vi "Example_Cursor.vi"() -> ()   [LabVIEW 2020, in "LcPictureBox.lvclass"]
uses:
  LcPictureBox.lvclass
  System.Windows.Forms
  SmoothingMode.ctl
  Pen.ctl
  CursorType.ctl
  ce328d88-1fef-4cb5-b4df-921596365a82.vi
  2765cc97-931e-4dce-9eb0-820734866045.vi
panel:
  in  "PictureBox 1":refnum<k24>(container)
  out "error out":errorcluster
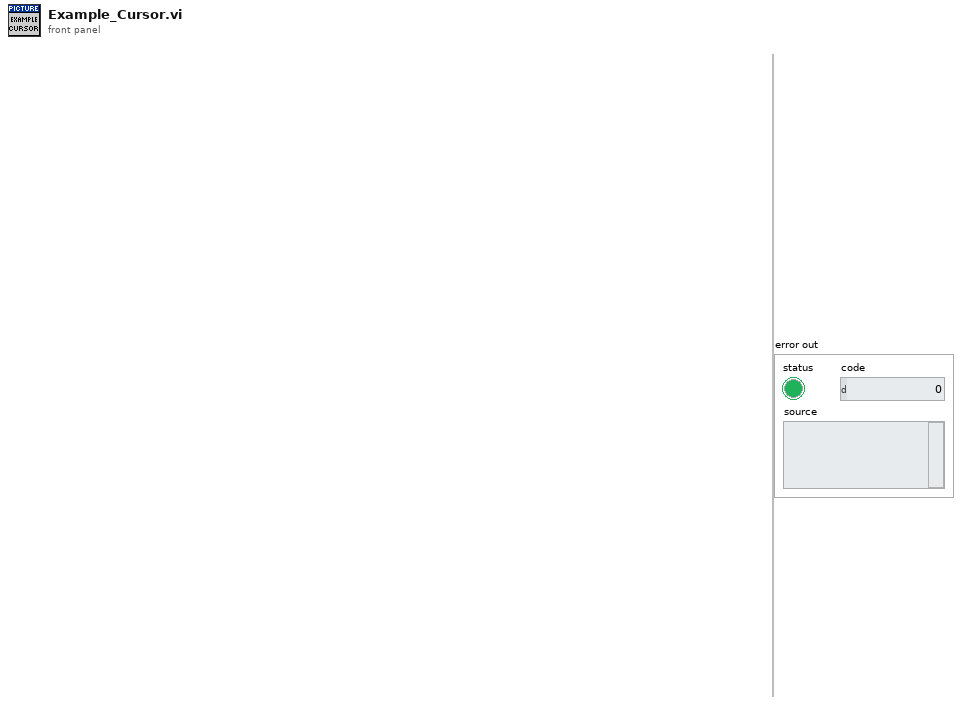
[diagram p1: front panel]
types:
  T1 = typedef "LcPictureBox.lvclass/CursorType.ctl" = enum16{"AppStarting", "Arrow", "Cross", "Default", "Hand", "Help", "HSplit", "IBeam", "No", "NoMove2D", "NoMoveHoriz", "NoMoveVert", "PanEast", "PanNE", "PanNorth", "PanNW", "PanSE", "PanSouth", "PanSW", "PanWest", "SizeAll", "SizeNESW", "SizeNS", "SizeNWSE", "SizeWE", "UpArrow", "VSplit", "WaitCursor"}
  T2 = typedef "LcPictureBox.lvclass/Pen.ctl" = cluster{"Width":u16, "Style":enum32{"Solid", "Dash", "Dot", "DashDot", "DashDotDot"}}
  T3 = typedef "LcPictureBox.lvclass/SmoothingMode.ctl" = enum16{"None", "HighSpeed", "HighQuality", "AntiAlias"}
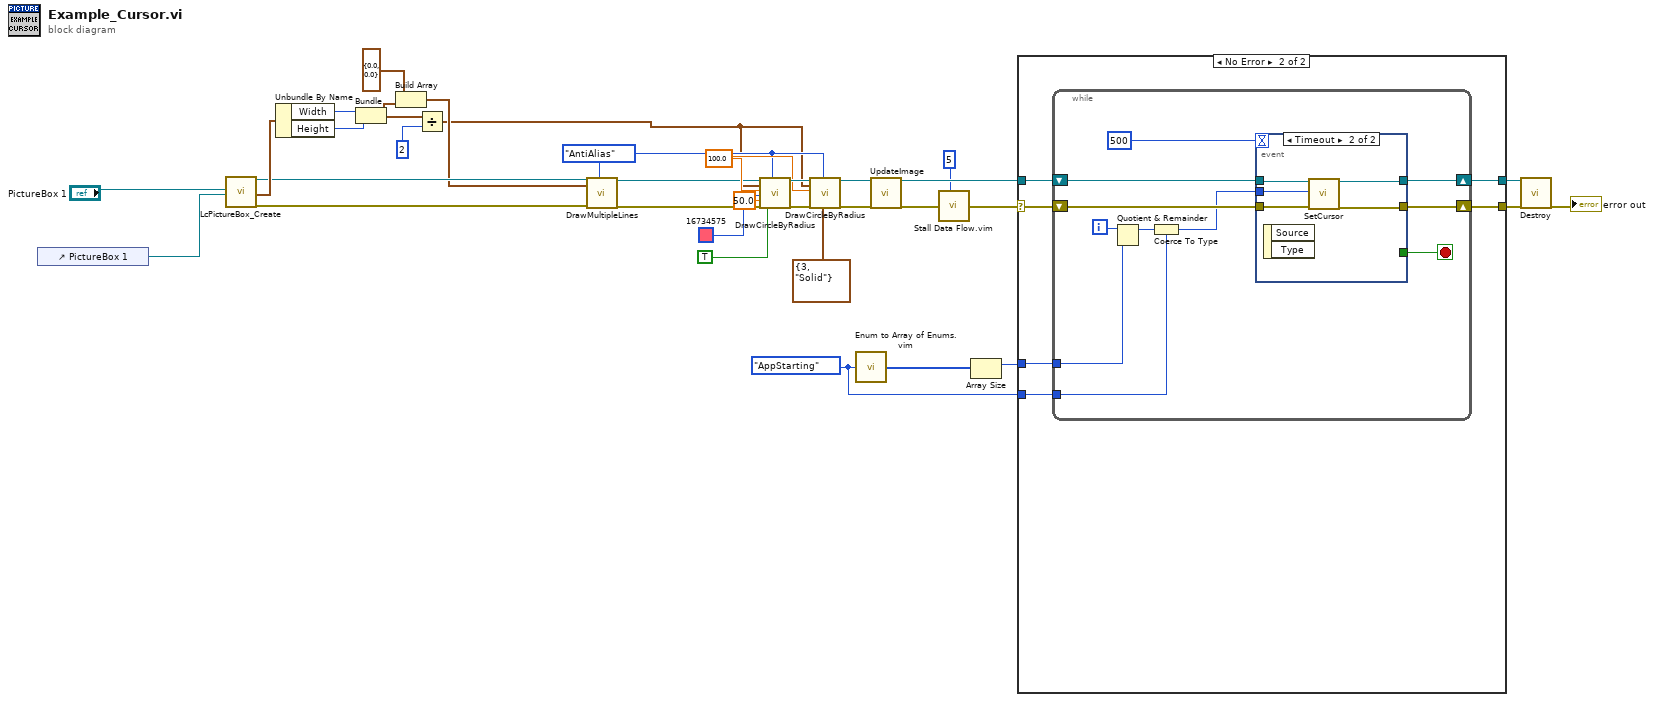
[diagram p0: block diagram]
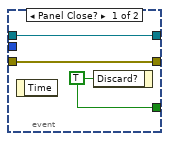
[diagram p3: hidden frame]
diagram:
  w2 = CursorType."AppStarting" ("CursorType")
  w10 = SmoothingMode."AntiAlias" ("SmoothingMode")
  w11 = sgl 100.0 ("Radius")
  n1 = control-ref of="PictureBox 1"() -> (w5:refnum<vi>)
  n2 = call "LcPictureBox_Create.vi"("PictureBox"="PictureBox 1", "PictureBoxActiveXReference"=w5) -> ("reference out"=w26:refnum<class "LcPictureBox.lvclass">, "ImageSizeUsed"=w34:cluster{"Width":i32, "Height":i32}, "Error Out"=w24:errorcluster)  [unwired: 15 in]
  n3 = Unbundle By Name(w34) -> ("Width"=w29:i32, "Height"=w28:i32)
  n4 = Bundle("Width"=w29, "Height"=w28) -> (w20:cluster{"Width":i32, "Height":i32})  [unwired: 1 in]
  n5 = Build Array(cluster{"x":dbl, "y":dbl} {"x"=0.0, "y"=0.0} ("Point"), w20) -> (w25:cluster{"x":dbl, "y":dbl}[])
  n6 = Divide(x=w20, y=2) -> (x/y=w7:cluster{"Width":dbl, "Height":dbl})
  n7 = call-dynamic "DrawMultipleLines.vi"("reference in"=w26, "LineEndPoints"=w25, "Error In"=w24, "SmoothingMode(AntiAlias)"=w10) -> ("reference out"=w8:refnum<class "LcPictureBox.lvclass">, "Error Out"=w9:errorcluster)  [unwired: 14 in]
  n8 = call-dynamic "DrawCircleByRadius.vi"("reference in"=w8, "Center"=w7, "Radius"=w11, "Color(Black)"=u32 16734575, "Alpha(100%)"=50.0, "Error In"=w9, "Fill(False)"=TRUE, "SmoothingMode(AntiAlias)"=w10) -> ("reference out"=w15:refnum<class "LcPictureBox.lvclass">, "Error Out"=w13:errorcluster)  [unwired: 10 in]
  n9 = call-dynamic "DrawCircleByRadius.vi"("reference in"=w15, "Center"=w7, "Radius"=w11, "Error In"=w13, "SmoothingMode(AntiAlias)"=w10, "Pen(Width=1, Solid)"=T2 {"Width"=3, "Style"=enum."Solid"}) -> ("reference out"=w14:refnum<class "LcPictureBox.lvclass">, "Error Out"=w12:errorcluster)  [unwired: 12 in]
  n10 = call "Enum to Array of Enums.vim"("enum"=w2) -> ("array of enums"=w4:T1[])
  n11 = call-dynamic "UpdateImage.vi"("reference in"=w14, "Error In"=w12) -> ("reference out"=w22:refnum<class "LcPictureBox.lvclass">, "Error Out"=w19:errorcluster)  [unwired: 14 in, 2 out]
  n12 = call "Stall Data Flow.vim"("value in"=w19, "milliseconds to wait"=u32 5 ("msToWait")) -> ("value out"=w21:errorcluster)  [unwired: 1 out]
  n13 = Array Size(array=w4) -> (size(s)=w3:i32)
  n14 = case shown="No Error" w21 {
    selector: w21 -> [w36 w39]
    tunnel: [w36 w42] -> w32
    tunnel: w22 -> [w35 w41]
    tunnel: [w35 w40] -> w31
    tunnel: w3 -> [_ w38]
    tunnel: w2 -> [_ w37]
    frame Error {
    }
    frame No Error {
      n15 = while {
        shift-right: [w51] -> w40
        shift-left: w41 -> [w52]
        shift-right: [w53] -> w42
        shift-left: w39 -> [w50]
        tunnel: w38 -> [w47]
        tunnel: w37 -> [w45]
        i -> [w44]
        stop <- w49 stop-if-true
        n16 = Quotient & Remainder(x=w44, y=w47) -> (x-y*floor(x/y)=w46:i32)  [unwired: 1 out]
        n17 = Coerce To Type(0:w46, 1:w45) -> (2:w43:T1)
        n18 = event shown="[1] Timeout" {
          selector: _ -> [_ _]
          dyn-events: _ -> [_ _]
          timeout: 500 -> [_ _]
          tunnel: w50 -> [w56 w60]
          tunnel: [w56 w59] -> w53
          tunnel: w52 -> [w55 w61]
          tunnel: [w55 w58] -> w51
          tunnel: [w54 _] -> w49
          tunnel: w43 -> [_ w57]
          event Panel Close? {
            w54 = TRUE ("Discard?")
            n19 = event-data() -> ()  [unwired: 1 in, 1 out]
            n20 = event-data("Discard?"=w54) -> ()  [unwired: 1 in, 1 out]
          }
          event Timeout {
            n21 = event-data() -> ()  [unwired: 1 in, 2 out]
            n22 = call-dynamic "SetCursor.vi"("reference in"=w61, "CursorType"=w57, "error in (no error)"=w60) -> ("reference out"=w58:refnum<class "LcPictureBox.lvclass">, "error out"=w59:errorcluster)  [unwired: 15 in]
          }
        }
      }
    }
  }
  n23 = call-dynamic "Destroy.vi"("reference in"=w31, "Error In"=w32) -> ("Error Out"=→"error out":errorcluster)  [unwired: 16 in, 1 out]
